vi "MCP2221_Input_Sample.vi"() -> ()   [LabVIEW 2025]
panel:
  out "GP3":bool
  out "GP2":bool
  out "GP1":bool
  out "GP0":bool
  out "error out":errorcluster
  in  "stop":bool
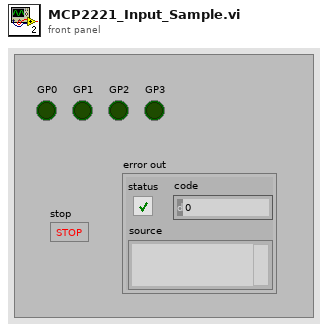
[diagram p1: front panel]
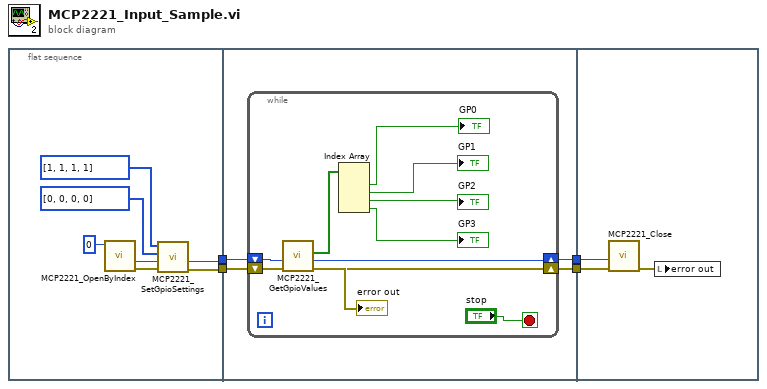
[diagram p0: block diagram]
diagram:
  n1 = flat-sequence {
    tunnel: [w8] -> w4
    tunnel: [w7] -> w3
    tunnel: w4 -> [w15]
    tunnel: w3 -> [w14]
    tunnel: [w13] -> w2
    tunnel: [w12] -> w1
    tunnel: w2 -> [w28]
    tunnel: w1 -> [w27]
    frame #0 {
      n2 = call "MCP2221_OpenByIndex.vi"("index"=u32 0) -> ("error out"=w10:errorcluster, "handle out"=w9:i32)  [unwired: 9 in]
      n3 = call "MCP2221_SetGpioSettings.vi"("error in"=w10, "handle in"=w9, "outputValues"=u8[] [0, 0, 0, 0], "pinDirections"=u8[] [1, 1, 1, 1]) -> ("error out"=w8:errorcluster, "handle out"=w7:i32)  [unwired: 5 in, 1 out]
    }
    frame #1 {
      n4 = while {
        shift-right: [w22] -> w12
        shift-left: w14 -> [w25]
        shift-right: [w23] -> w13
        shift-left: w15 -> [w24]
        stop <- "stop" stop-if-true
        n5 = call "MCP2221_GetGpioValues.vi"("error in"=w24, "handle in"=w25) -> ("error out"=w23:errorcluster, "handle out"=w22:i32, "gpio"=w20:bool[])  [unwired: 6 in, 1 out]
        n6 = Index Array(array=w20) -> (element #1=→"GP0":bool, element #2=→"GP1":bool, element #3=→"GP2":bool, element #4=→"GP3":bool)  [unwired: 4 in]
        "error out" <- w24
      }
    }
    frame #2 {
      n7 = call "MCP2221_Close.vi"("error in"=w28, "handle in"=w27) -> ("error out"=w26:errorcluster)  [unwired: 7 in, 2 out]
      n8 = local write "error out"(w26) -> ()
    }
  }
